vi "DOE Check Power Thresholds.vi"(7 "Power (W):Sigma":dbl, 8 "Error In":errorcluster, 9 "Power Limit (Watts)":dbl, 10 "Wait for Power Threshold":bool) -> (0 "Error Out":errorcluster, 2 "Wait for Power Threshold (Output)":bool, 3 "States":string)   [LabVIEW 2016]
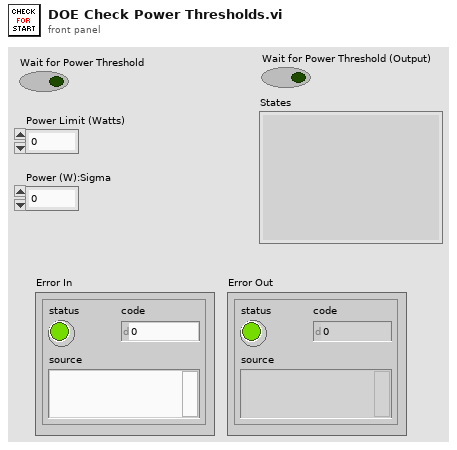
[diagram p1: front panel]
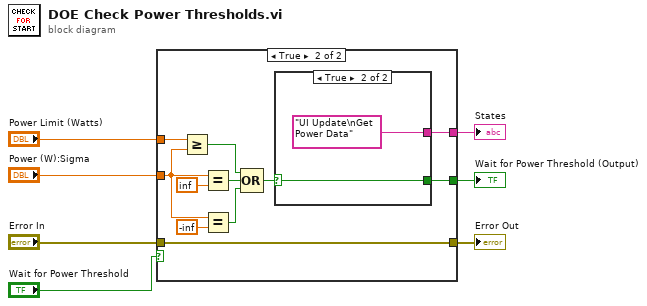
[diagram p0: block diagram]
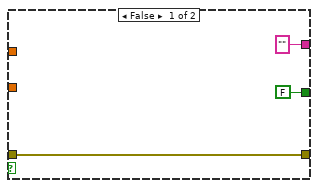
[diagram p2: hidden frame]
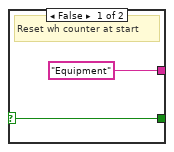
[diagram p3: hidden frame]
diagram:
  n1 = case shown="True" "Wait for Power Threshold" {
    tunnel: [FALSE w18] -> w6
    tunnel: "Power Limit (Watts)" -> [_ w21]
    tunnel: "Power (W):Sigma" -> [_ w17]
    tunnel: ["" w20] -> w5
    tunnel: "Error In" -> [w8 w19]
    tunnel: [w8 w19] -> w1
    frame False {
    }
    frame True {
      n2 = Greater Or Equal?(x=w21, y=w17) -> (x >= y?=w12:bool)
      n3 = Equal?(x=w17, y=inf) -> (x = y?=w14:bool)
      n4 = Equal?(x=w17, y=-inf) -> (x = y?=w13:bool)
      n5 = Compound Arithmetic op=OR(w12, w14, w13) -> (w11:bool)
      n6 = case shown="True" w11 {
        selector: w11 -> [w22 w24]
        tunnel: ["Equipment" "UI Update\nGet Power Data"] -> w20
        tunnel: [w22 w24] -> w18
        frame False {
          # "Reset wh counter at start"
        }
        frame True {
        }
      }
    }
  }
  "Wait for Power Threshold (Output)" <- w6
  "States" <- w5
  "Error Out" <- w1
